vi "smartmeshIP stress testing.vi"(6 "mac adresses":T1, 7 "stress testing enabled":bool, 8 "error in":errorcluster, 9 "last packet type dust":i32[](array[numeric]), 10 "last packet type ngi":u8[](array[numeric]), 11 "Adjustable Parameters":T2(array[cluster]) {"ACMP0 ch" items=["Geophone 1"=0, "Geophone 2"=3, "Geophone 3"=4, "Geophone 4"=5]; "ACMP1 ch" items=["Geophone 2"=1, "Geophone 3"=2, "Geophone 4"=3]}) -> (0 "error out":errorcluster)   [LabVIEW 2017]
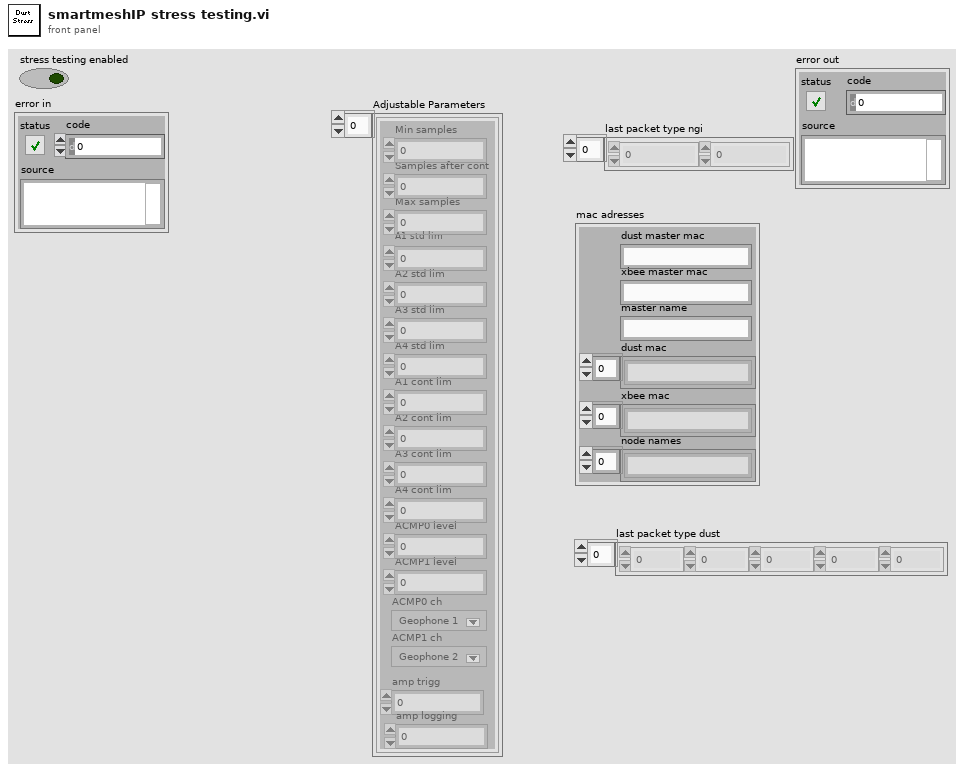
[diagram p1: front panel]
types:
  T1 = cluster{"dust master mac":string, "xbee master mac":string, "master name":string, "dust mac":string[], "xbee mac":string[], "node names":string[]}
  T2 = cluster{"Min samples":u32, "Samples after cont":u32, "Max samples":u32, "A1 std lim":sgl, "A2 std lim":sgl, "A3 std lim":sgl, "A4 std lim":sgl, "A1 cont lim":sgl, "A2 cont lim":sgl, "A3 cont lim":sgl, "A4 cont lim":sgl, "ACMP0 level":u32, "ACMP1 level":u32, "ACMP0 ch":u8, "ACMP1 ch":u8, "amp trigg":u16, "amp logging":u16}[]
  T3 = typedef "LVDateTimeRec.ctl" = cluster{"fractional second":dbl, "second":i32, "minute":i32, "hour":i32, "day of month":i32, "month":i32, "year":i32, "day of week":i32, "day of year":i32, "DST":i32}
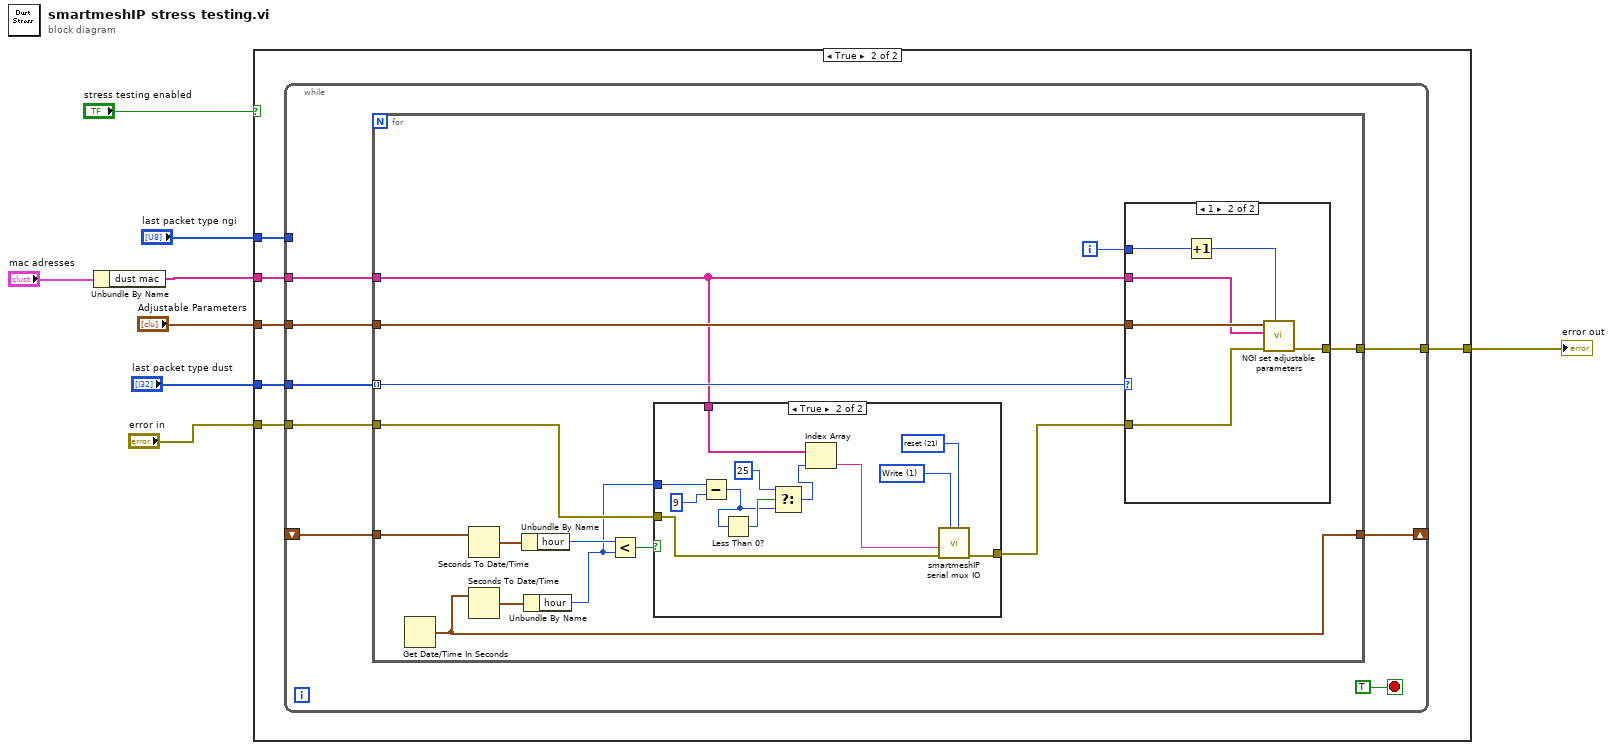
[diagram p0: block diagram]
diagram:
  n1 = Unbundle By Name("mac adresses") -> ("dust mac"=w5:string[])
  n2 = case shown="True" "stress testing enabled" {
    tunnel: "last packet type ngi" -> [_ w15]
    tunnel: "Adjustable Parameters" -> [_ w14]
    tunnel: w5 -> [_ w13]
    tunnel: "last packet type dust" -> [_ w12]
    tunnel: "error in" -> [w9 w11]
    tunnel: [w9 w10] -> w1
    frame False {
    }
    frame True {
      n3 = while {
        tunnel: w15 -> [_]
        tunnel: w13 -> [w19]
        tunnel: w14 -> [w22]
        tunnel: w12 -> [w18]
        tunnel: w11 -> [w21]
        tunnel: [w20] -> w10
        shift-right: [w17] -> _
        shift-left: _ -> [w16]
        stop <- TRUE stop-if-true
        n4 = for {
          tunnel: w19 -> [w26]
          tunnel: w22 -> [w36]
          tunnel: w18 -> [w37] mode=indexing
          tunnel: w21 -> [w28]
          tunnel: [w35] -> w20
          tunnel: [w32] -> w17
          tunnel: w16 -> [w33]
          i -> [w34]
          n5 = Get Date/Time In Seconds() -> (seconds since 1Jan1904=w32:timestamp)
          n6 = Seconds To Date/Time(time stamp (now)=w33) -> (date time rec=w31:T3)  [unwired: 1 in]
          n7 = Seconds To Date/Time(time stamp (now)=w32) -> (date time rec=w30:T3)  [unwired: 1 in]
          n8 = Unbundle By Name(w31) -> ("hour"=w25:i32)
          n9 = Unbundle By Name(w30) -> ("hour"=w24:i32)
          n10 = Less?(x=w25, y=w24) -> (x < y?=w29:bool)
          n11 = case shown="True" w29 {
            tunnel: w28 -> [w38 w50]
            tunnel: [w38 w49] -> w27
            tunnel: w26 -> [_ w41]
            tunnel: w24 -> [_ w42]
            frame False {
            }
            frame True {
              w47 = u8 21 items=["subscribe"=22, "startNetwork"=45, "setUser"=58, "setTime"=54, "setNetworkConfig"=26, "setLicense"=56, "setIPConfig"=68, "setDownstreamFrameMode"=51, "setCommonJoinKey"=66, "setAdvertising"=50, "setACLEntry"=39, "sendIP"=59, "sendData"=44, "restorFactoryDefaults"=61, "reset"=21, "radiotestTx"=35, "radiotestRx"=37, "pingMote"=42, "getTime"=23, "getSystemInfo"=46, "radiotestStatistics"=38, "getPathInfo"=48, "getNextPath"=49, "getNextACLEntry"=40, "getNetworkInfo"=64, "getNetworkConfig"=63, "getMoteLinks"=70, "getMoteInfo"=62, "getMoteConfigByld"=65, "getMoteConfig"=47, "getManagerStatistics"=53, "getLog"=43, "getLicense"=55, "getIPConfig"=67, "exchangeNetworkID"=34, "exchangeMoteJoinKey"=33, "deleteMote"=69, "deleteACLEntry"=41, "clearStatistics"=31] ("tx_commandType")
              w48 = u16 1 items=["Connect", "Write", "Read", "Close"] ("State")
              n12 = Subtract(x=w42, y=9) -> (x-y=w39:i32)
              n13 = Less Than 0?(x=w39) -> (x < 0?=w43:bool)
              n14 = Select(t=25 ("f"), s=w43, f=w39) -> (s? t:f=w44:i32)
              n15 = Index Array(array=w41, index=w44) -> (element=w46:string)
              n16 = call "smartmeshIP serial mux IO.vi"("tx_commandType"=w47, "State"=w48, "error in"=w50, "MAC source"=w46) -> ("error out"=w49:errorcluster)  [unwired: 2 in, 5 out]
            }
          }
          n17 = case shown="1" w37 {
            tunnel: w36 -> [_ w57]
            tunnel: w34 -> [_ w56]
            tunnel: w26 -> [_ w54]
            tunnel: w27 -> [w51 w53]
            tunnel: [w51 w52] -> w35
            frame 0, Default {
            }
            frame 1 {
              n18 = Increment(x=w56) -> (x+1=w55:i32)
              n19 = call "NGI set adjustable parameters.vi"("node nummer"=w55, "error in"=w53, "dust mac adress"=w54, "Adjustable Parameters"=w57) -> ("error out"=w52:errorcluster)  [unwired: 7 in]
            }
          }
        }
      }
    }
  }
  "error out" <- w1
